vi "Untitled 330.vi"(2 "Error In":errorcluster, 3 "filename":string="D:/amarcos/Documentos/JRipoll/ScanCube/scancube_jaguirre/gridscancube/Correction Files/Cor_1to1.ctb") -> (0 "Error Out":errorcluster, 1 "String":string)   [LabVIEW 2015]
uses:
  <vilib>/Utility/error.llb/DialogType.ctl
  <userlib>/SCANalone4x64/SCANalone4x64.lvlib
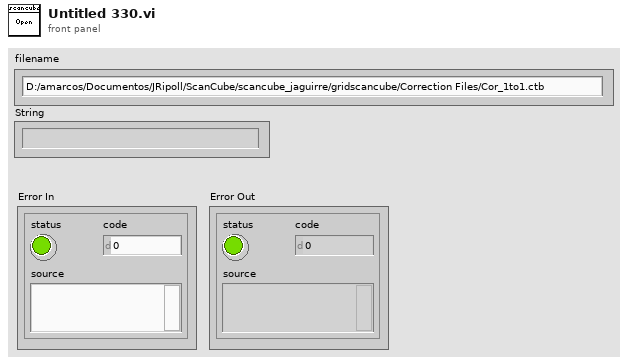
[diagram p1: front panel]
types:
  T1 = typedef "DialogType.ctl" = u16
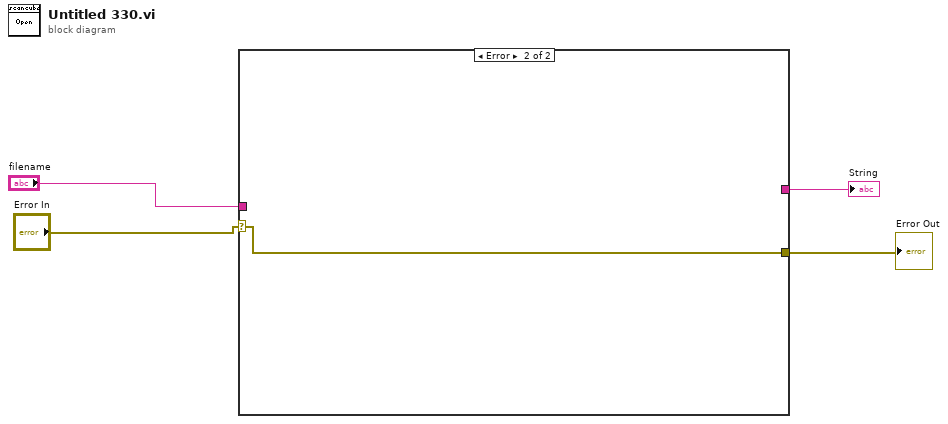
[diagram p0: block diagram]
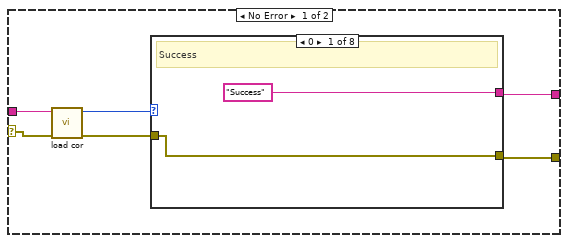
[diagram p2: hidden frame]
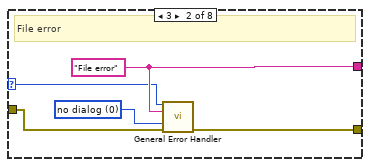
[diagram p3: hidden frame]
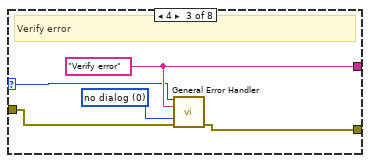
[diagram p4: hidden frame]
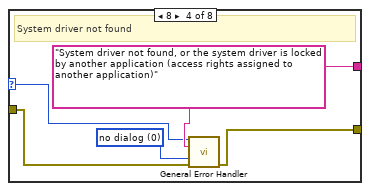
[diagram p5: hidden frame]
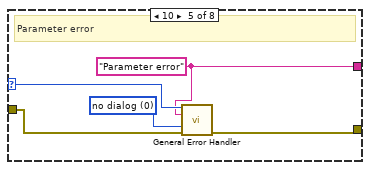
[diagram p6: hidden frame]
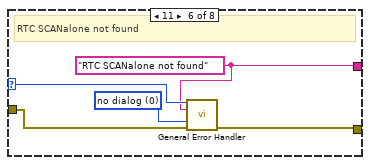
[diagram p7: hidden frame]
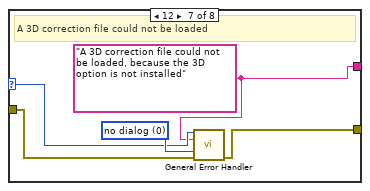
[diagram p8: hidden frame]
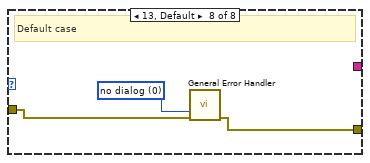
[diagram p9: hidden frame]
diagram:
  n1 = case shown="Error" "Error In" {
    selector: "Error In" -> [w5 w46]
    tunnel: "filename" -> [w10 _]
    tunnel: [w8 _] -> w3
    tunnel: [w6 w46] -> w2
    frame No Error {
      n2 = call <userlib>:"load cor.vi"("error in (no error)"=w5, "filename"=w10) -> ("error out"=w7:errorcluster, "function return"=w9:i16)  [unwired: 8 in]
      n3 = case shown="0" w9 {
        selector: w9 -> [_ w13 w18 w23 w30 w35 w40 _]
        tunnel: ["Success" w14 w19 w24 w29 w34 w39 _] -> w8
        tunnel: w7 -> [w11 w16 w21 w26 w31 w36 w41 w44]
        tunnel: [w11 w15 w20 w25 w28 w33 w38 w43] -> w6
        frame 0 {
          # "Success"
        }
        frame 3 {
          w17 = T1 0 items=["no dialog", "OK message", "continue or stop message", "OK message + warnings", "continue/stop + warnings"] ("type of dialog (OK msg:1)")
          w14 = "File error"
          # "File error"
          n4 = call <vilib>:"General Error Handler.vi"("[error code] (0)"=w13, "[error source] (\" \")"=w14, "type of dialog (OK msg:1)"=w17, "error in (no error)"=w16) -> ("error out"=w15:errorcluster)  [unwired: 7 in, 4 out]
        }
        frame 4 {
          w22 = T1 0 items=["no dialog", "OK message", "continue or stop message", "OK message + warnings", "continue/stop + warnings"] ("type of dialog (OK msg:1)")
          w19 = "Verify error"
          # "Verify error"
          n5 = call <vilib>:"General Error Handler.vi"("[error code] (0)"=w18, "[error source] (\" \")"=w19, "type of dialog (OK msg:1)"=w22, "error in (no error)"=w21) -> ("error out"=w20:errorcluster)  [unwired: 7 in, 4 out]
        }
        frame 8 {
          w27 = T1 0 items=["no dialog", "OK message", "continue or stop message", "OK message + warnings", "continue/stop + warnings"] ("type of dialog (OK msg:1)")
          w24 = "System driver not found, or the system driver is locked by another application (access rights assigned to another application)"
          # "System driver not found"
          n6 = call <vilib>:"General Error Handler.vi"("[error code] (0)"=w23, "[error source] (\" \")"=w24, "type of dialog (OK msg:1)"=w27, "error in (no error)"=w26) -> ("error out"=w25:errorcluster)  [unwired: 7 in, 4 out]
        }
        frame 10 {
          w32 = T1 0 items=["no dialog", "OK message", "continue or stop message", "OK message + warnings", "continue/stop + warnings"] ("type of dialog (OK msg:1)")
          w29 = "Parameter error"
          # "Parameter error"
          n7 = call <vilib>:"General Error Handler.vi"("[error code] (0)"=w30, "[error source] (\" \")"=w29, "type of dialog (OK msg:1)"=w32, "error in (no error)"=w31) -> ("error out"=w28:errorcluster)  [unwired: 7 in, 4 out]
        }
        frame 11 {
          w37 = T1 0 items=["no dialog", "OK message", "continue or stop message", "OK message + warnings", "continue/stop + warnings"] ("type of dialog (OK msg:1)")
          w34 = "RTC SCANalone not found"
          # "RTC SCANalone not found"
          n8 = call <vilib>:"General Error Handler.vi"("[error code] (0)"=w35, "[error source] (\" \")"=w34, "type of dialog (OK msg:1)"=w37, "error in (no error)"=w36) -> ("error out"=w33:errorcluster)  [unwired: 7 in, 4 out]
        }
        frame 12 {
          w42 = T1 0 items=["no dialog", "OK message", "continue or stop message", "OK message + warnings", "continue/stop + warnings"] ("type of dialog (OK msg:1)")
          w39 = "A 3D correction file could not be loaded, because the 3D option is not installed"
          # "A 3D correction file could not be loaded"
          n9 = call <vilib>:"General Error Handler.vi"("[error code] (0)"=w40, "[error source] (\" \")"=w39, "type of dialog (OK msg:1)"=w42, "error in (no error)"=w41) -> ("error out"=w38:errorcluster)  [unwired: 7 in, 4 out]
        }
        frame 13, Default {
          w45 = T1 0 items=["no dialog", "OK message", "continue or stop message", "OK message + warnings", "continue/stop + warnings"] ("type of dialog (OK msg:1)")
          # "Default case"
          n10 = call <vilib>:"General Error Handler.vi"("type of dialog (OK msg:1)"=w45, "error in (no error)"=w44) -> ("error out"=w43:errorcluster)  [unwired: 9 in, 4 out]
        }
      }
    }
    frame Error {
    }
  }
  "String" <- w3
  "Error Out" <- w2
